vi "Get_Day_File_Client.vi"(4 "Averaging Time (min)":dbl=5.0, 5 "End time":timestamp, 6 "Start time":timestamp, 7 "Channel Names":string[](array[string]), 8 "Data folder location":path=path "/G4-2-HD/Enflo Data/Server Day Files") -> (0 "Files with wrong times":path[](array[path]), 1 "All Channel Names":string[](array[string]), 2 "Data":dbl[][](array[numeric]), 3 "Times":dbl[](array[numeric]))   [LabVIEW 2010]
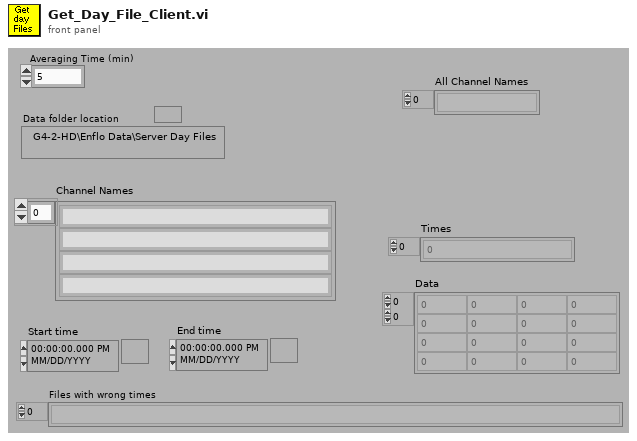
[diagram p1: front panel]
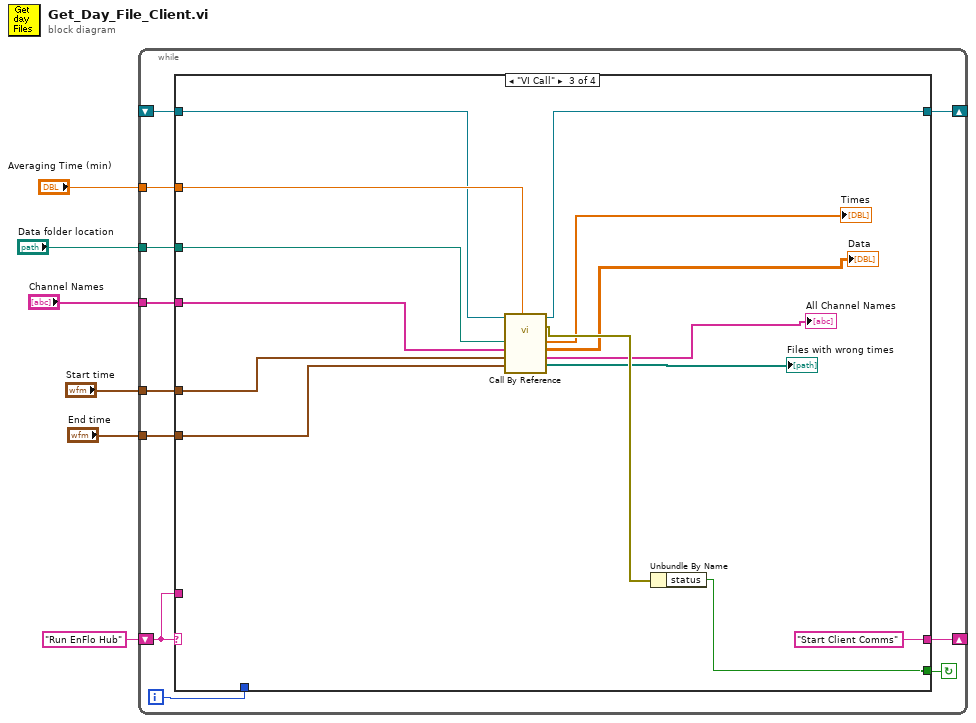
[diagram p0: block diagram]
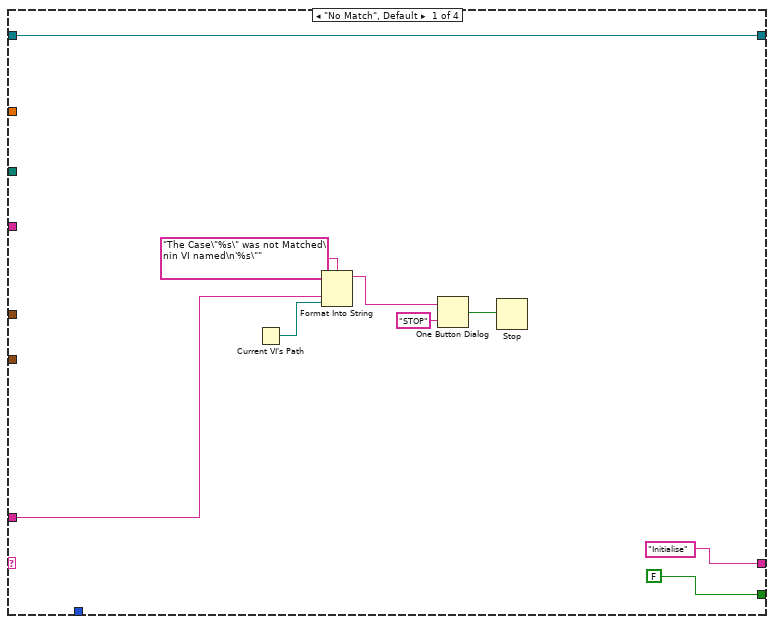
[diagram p2: hidden frame]
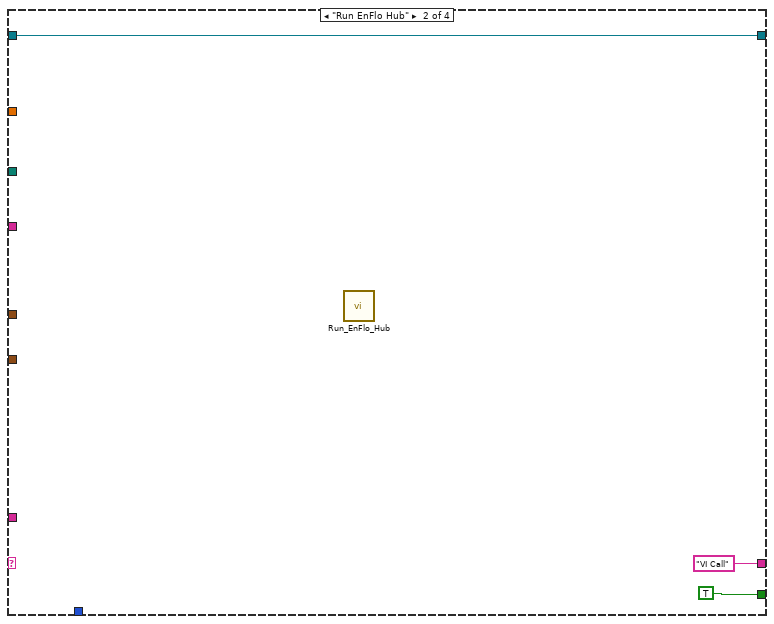
[diagram p3: hidden frame]
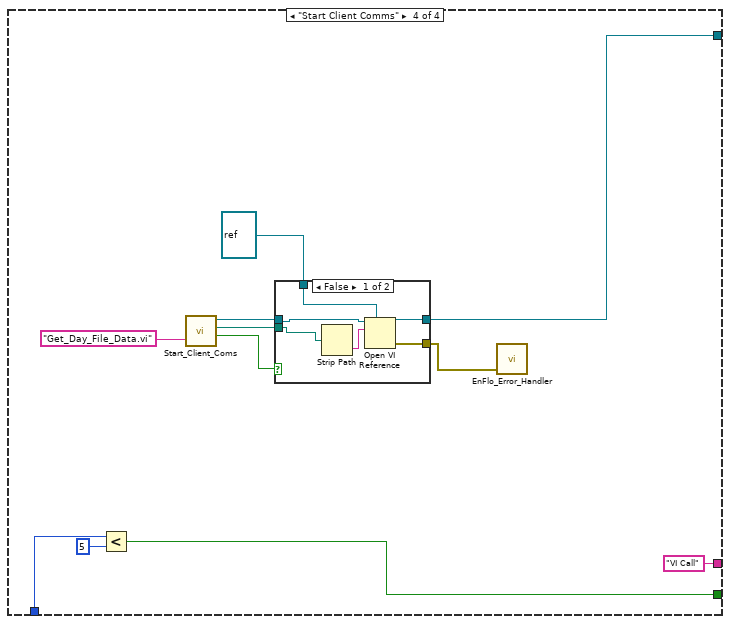
[diagram p4: hidden frame]
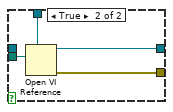
[diagram p5: hidden frame]
diagram:
  n1 = while {
    shift-left: "Run EnFlo Hub" -> [w15]
    shift-right: [w16] -> _
    shift-right: [w9] -> _
    shift-left: _ -> [w8]
    tunnel: "Data folder location" -> [w14]
    tunnel: "Channel Names" -> [w13]
    tunnel: "Start time" -> [w12]
    tunnel: "End time" -> [w11]
    tunnel: "Averaging Time (min)" -> [w10]
    i -> [w7]
    stop <- w17 continue-if-true
    n2 = case shown="\"VI Call\"" w15 {
      tunnel: [FALSE TRUE w36 w44] -> w17
      tunnel: ["Initialise" "VI Call" "Start Client Comms" "VI Call"] -> w16
      tunnel: w15 -> [w21 _ _ _]
      tunnel: w14 -> [_ _ w42 _]
      tunnel: w13 -> [_ _ w41 _]
      tunnel: w12 -> [_ _ w40 _]
      tunnel: w11 -> [_ _ w39 _]
      tunnel: w10 -> [_ _ w38 _]
      tunnel: [w18 w28 w30 w49] -> w9
      tunnel: w8 -> [w18 w28 w31 _]
      tunnel: w7 -> [_ _ _ w46]
      frame "No Match", Default {
        n3 = Current VI's Path() -> (path=w20:path)
        n4 = Format Into String(format string="The Case\"%s\" was not Matched\nin VI named\n'%s\"" ("Format String"), w21, w20) -> (resulting string=w24:string)  [unwired: 2 in, 1 out]
        n5 = One Button Dialog(message=w24, button name ("OK")="STOP") -> (true=w22:bool)
        n6 = Stop(stop? (T)=w22) -> ()
      }
      frame "Run EnFlo Hub" {
        n7 = call "Run_EnFlo_Hub.vi"() -> ()  [unwired: 8 out]
      }
      frame "VI Call" {
        n8 = call-by-ref "?"(reference=w31, "Averaging Time (min)"=w38, "End time"=w39, "Start time"=w40, "Channel Names"=w41, "Data folder location"=w42) -> (reference out=w30:refnum<vi>, error out=w37:errorcluster, "Files with wrong times"=→"Files with wrong times":path[], "All Channel Names"=→"All Channel Names":string[], "Data"=→"Data":dbl[][], "Times"=→"Times":dbl[])  [unwired: 1 in]
        n9 = Unbundle By Name(w37) -> ("status"=w36:bool)
      }
      frame "Start Client Comms" {
        n10 = Less?(x=w46, y=5) -> (x < y?=w44:bool)
        n11 = call "Start_Client_Coms.vi"("VI name to run on server"="Get_Day_File_Data.vi") -> ("LabVIEW application reference"=w52:refnum<vi>, "Checked VI name"=w54:path, "Local Call"=w53:bool)  [unwired: 1 in, 1 out]
        n12 = case shown="False" w53 {
          tunnel: refnum<vi> refnum ("trivial.vi type") -> [w56 w64]
          tunnel: w54 -> [w57 w63]
          tunnel: w52 -> [w55 _]
          tunnel: [w59 w62] -> w48
          tunnel: [w58 w61] -> w49
          frame False {
            n13 = Strip Path(path=w57) -> (name=w60:string)  [unwired: 1 out]
            n14 = Open VI Reference(type specifier VI Refnum (for type only)=w56, application reference (local)=w55, vi path=w60) -> (vi reference=w58:refnum<vi>, error out=w59:errorcluster)  [unwired: 1 in, 2 out]
          }
          frame True {
            n15 = Open VI Reference(type specifier VI Refnum (for type only)=w64, vi path=w63) -> (vi reference=w61:refnum<vi>, error out=w62:errorcluster)  [unwired: 1 in, 3 out]
          }
        }
        n16 = call "EnFlo_Error_Handler.vi"("error in (no error)"=w48) -> ()  [unwired: 2 in, 3 out]
      }
    }
  }
